vi "test_libssh2_session_handshake.vi"() -> ()   [LabVIEW 2017, in "integration_tests.lvlib"]
uses:
  integration_tests.lvlib
  libssh2/libssh2_session_handshake_tcp.vi
  libssh2/libssh2_init_default.vi
  libssh2/libssh2_session_init_ex.vi
  <vilib>/Utility/tcp.llb/TCP Get Raw Net Object.vi
  libssh2/libssh2_session_handshake_socket.vi
  libssh2/libssh2.lvlib
  support/support.lvlib
  <vilib>/PNR/Transparent Assertions/Transparent Assertions/Transparent Assertions.lvlib
panel:
  out "error out":errorcluster
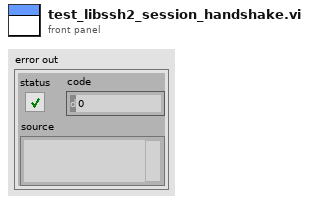
[diagram p1: front panel]
types:
  T1 = typedef "libssh2.lvlib/Session Refnum.ctl" = refnum<k1>
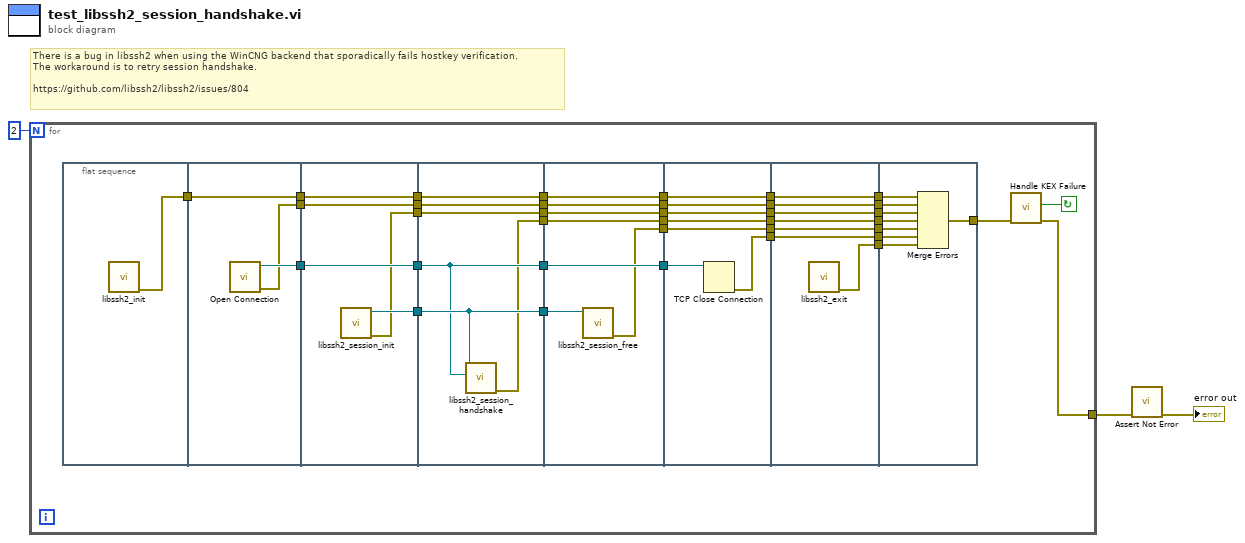
[diagram p0: block diagram]
diagram:
  # "There is a bug in libssh2 when using the WinCNG backend that sporadically fails hostkey verification.\nThe workaround is to retry session handshake.\n\nhttps://github.com/libssh2/libssh2/issues/804"
  n1 = for {
    N: 2 -> [_]
    tunnel: [w8] -> w2
    stop <- w9 continue-if-true
    n2 = flat-sequence {
      tunnel: [w41] -> w40
      tunnel: [w44] -> w39
      tunnel: w40 -> [w43]
      tunnel: [w43] -> w38
      tunnel: [w42] -> w37
      tunnel: w39 -> [w49]
      tunnel: [w49] -> w36
      tunnel: w38 -> [w48]
      tunnel: [w48] -> w35
      tunnel: w37 -> [w47]
      tunnel: [w47] -> w34
      tunnel: [w46] -> w33
      tunnel: [w45] -> w32
      tunnel: w36 -> [w51]
      tunnel: [w51] -> w31
      tunnel: w35 -> [w55]
      tunnel: [w55] -> w30
      tunnel: w34 -> [w54]
      tunnel: [w54] -> w29
      tunnel: [w53] -> w28
      tunnel: w33 -> [w53]
      tunnel: w32 -> [w52]
      tunnel: [w52] -> w27
      tunnel: [w50] -> w7
      tunnel: w31 -> [w62]
      tunnel: [w62] -> w26
      tunnel: w30 -> [w61]
      tunnel: [w61] -> w25
      tunnel: w29 -> [w60]
      tunnel: [w60] -> w24
      tunnel: w28 -> [w59]
      tunnel: w27 -> [w58]
      tunnel: [w58] -> w23
      tunnel: [w57] -> w22
      tunnel: w7 -> [w56]
      tunnel: [w56] -> w6
      tunnel: w26 -> [w69]
      tunnel: w25 -> [w68]
      tunnel: [w68] -> w21
      tunnel: w24 -> [w67]
      tunnel: [w67] -> w20
      tunnel: [w66] -> w19
      tunnel: w23 -> [w65]
      tunnel: [w65] -> w18
      tunnel: w22 -> [w64]
      tunnel: [w64] -> w17
      tunnel: w6 -> [w63]
      tunnel: [w63] -> w5
      tunnel: w21 -> [w76]
      tunnel: [w76] -> w16
      tunnel: w20 -> [w75]
      tunnel: [w75] -> w15
      tunnel: w19 -> [w74]
      tunnel: [w74] -> w14
      tunnel: [w73] -> w13
      tunnel: w18 -> [w72]
      tunnel: [w72] -> w12
      tunnel: w17 -> [w71]
      tunnel: [w71] -> w11
      tunnel: w5 -> [w70]
      tunnel: [w70] -> w4
      tunnel: w16 -> [w84]
      tunnel: w15 -> [w83]
      tunnel: w14 -> [w82]
      tunnel: w13 -> [w81]
      tunnel: w12 -> [w80]
      tunnel: w11 -> [w79]
      tunnel: [w78] -> w10
      tunnel: w4 -> [w77]
      frame #0 {
        n3 = call-poly "libssh2_init.vi"() -> ("error out"=w41:errorcluster)  [unwired: 11 in]
      }
      frame #1 {
        n4 = call "Open Connection.vi"() -> ("error out"=w42:errorcluster, "connection ID"=w44:refnum<k5>)  [unwired: 10 in]
      }
      frame #2 {
        n5 = call "libssh2_session_init.vi"() -> ("error out"=w45:errorcluster, "session"=w46:T1)  [unwired: 10 in]
      }
      frame #3 {
        n6 = call-poly "libssh2_session_handshake.vi"("tcp connection"=w51, "session"=w53) -> ("error out"=w50:errorcluster)  [unwired: 9 in]
      }
      frame #4 {
        n7 = call "libssh2_session_free.vi"("session"=w59) -> ("error out"=w57:errorcluster)  [unwired: 10 in]
      }
      frame #5 {
        n8 = TCP Close Connection(connection ID=w69) -> (error out=w66:errorcluster)  [unwired: 2 in, 1 out]
      }
      frame #6 {
        n9 = call "libssh2_exit.vi"() -> ("error out"=w73:errorcluster)  [unwired: 11 in]
      }
      frame #7 {
        n10 = Merge Errors(w84, w83, w80, w77, w79, w82, w81) -> (w78:errorcluster)
      }
    }
    n11 = call "Handle KEX Failure.vi"("error in (no error)"=w10) -> ("error out"=w8:errorcluster, "KEX Failure"=w9:bool)  [unwired: 9 in]
  }
  n12 = call <vilib>:"Assert Not Error.vi"("error in (no error)"=w2) -> ("error out"=→"error out":errorcluster)  [unwired: 10 in]
